vi "Set_Coupling.vi"(4 "Status":i32, 5 "error in (no error)":errorcluster, 6 "Set Coupling":u16(ring) items=["AC", "DC"], 7 "Choose_Device":T1(ring), 8 "Index":i32) -> (0 "error out":errorcluster, 1 "Status_out":i32, 2 "Device_type":T1(ring), 3 "Index_Out":i32)   [LabVIEW 2013, in "FEMTO_LUCI-10.lvlib"]
doc: "This function sets AC/DC coupling for the selected device."
uses:
  FEMTO_LUCI-10.lvlib
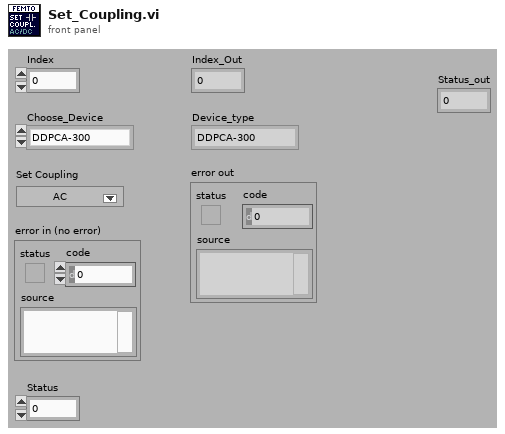
[diagram p1: front panel]
types:
  T1 = enum16{"DDPCA-300", "DLPCA-200", "DHPCA-100", "OE-200", "LIA-MV-150-S", "LIA-MV-150-D", "LIA-MV-200-L", "LIA-MV-200-H", "LIA-MVD-200-L", "LIA-MVD-200-H", "DLPVA-100-BUN-S", "DLPVA-100-BLN-S", "DLPVA-100-B-S", "DLPVA-100-B-D", "DLPVA-100-F-S", "DLPVA-100-F-D", "DHPVA-100", "DHPVA-200", "DUPVA-1-60", "DUPVA-1-70"}
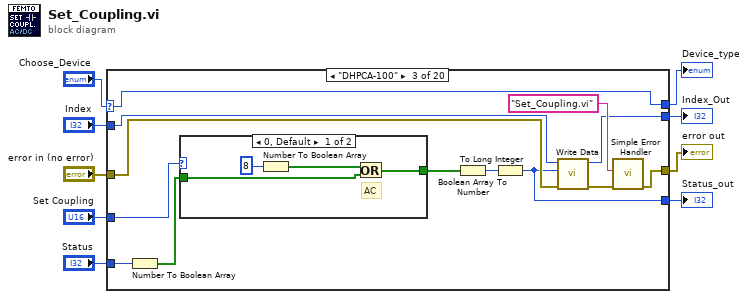
[diagram p0: block diagram]
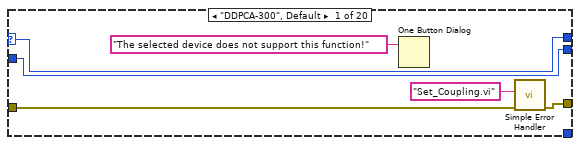
[diagram p2: hidden frame]
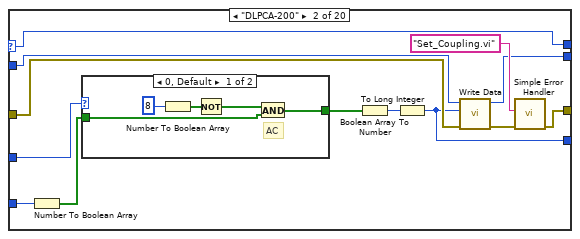
[diagram p3: hidden frame]
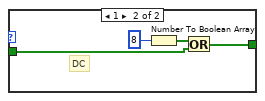
[diagram p4: hidden frame]
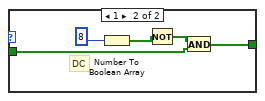
[diagram p5: hidden frame]
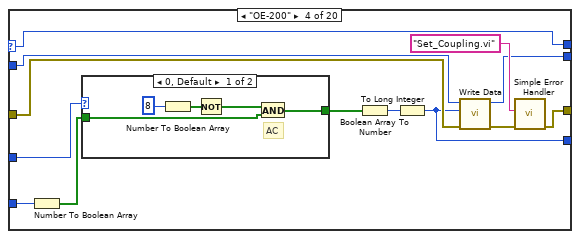
[diagram p6: hidden frame]
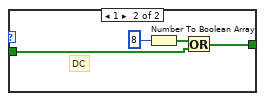
[diagram p7: hidden frame]
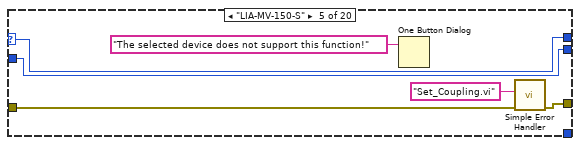
[diagram p8: hidden frame]
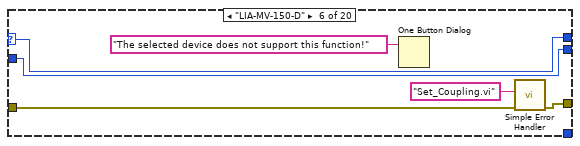
[diagram p9: hidden frame]
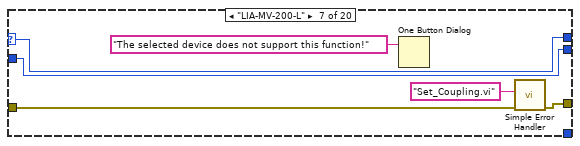
[diagram p10: hidden frame]
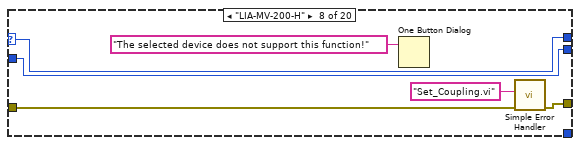
[diagram p11: hidden frame]
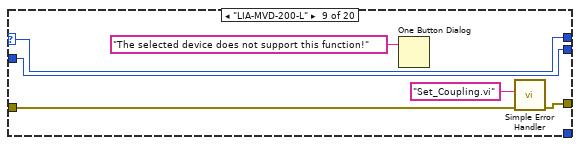
[diagram p12: hidden frame]
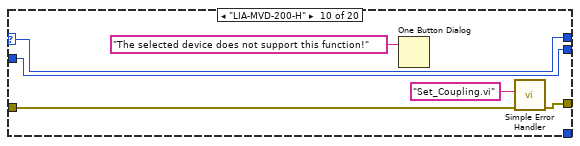
[diagram p13: hidden frame]
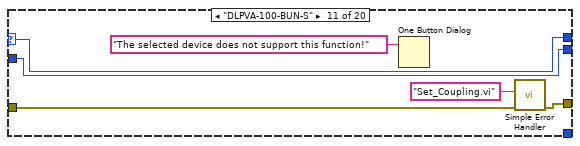
[diagram p14: hidden frame]
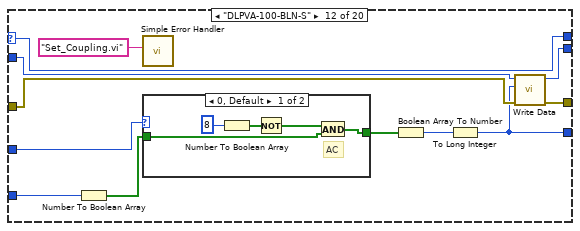
[diagram p15: hidden frame]
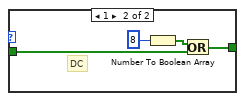
[diagram p16: hidden frame]
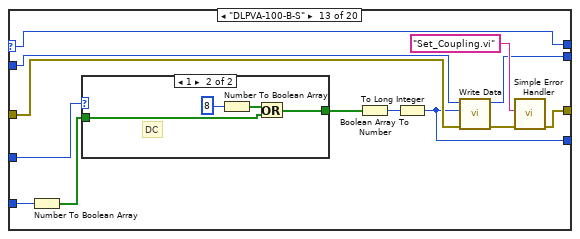
[diagram p17: hidden frame]
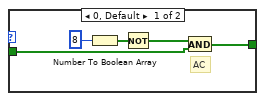
[diagram p18: hidden frame]
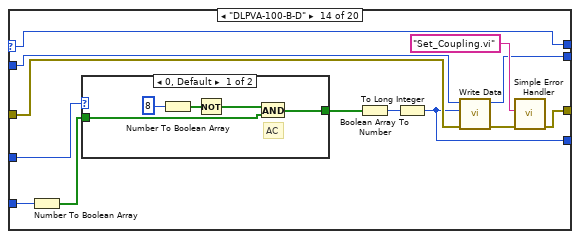
[diagram p19: hidden frame]
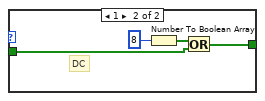
[diagram p20: hidden frame]
diagram:
  n1 = case shown="\"DHPCA-100\"" "Choose_Device" {
    selector: "Choose_Device" -> [w13 w27 w48 w70 w85 w91 w97 w103 w109 w115 w121 w134 w155 w172 w200 w221 w243 w265 w279 w285]
    tunnel: "error in (no error)" -> [w12 w18 w40 w62 w83 w89 w95 w102 w106 w112 w120 w130 w149 w174 w193 w215 w239 w261 w281 w287]
    tunnel: [w14 w28 w50 w71 w86 w92 w98 w104 w110 w116 w122 w129 w156 w178 w199 w222 w244 w266 w280 w286] -> w4
    tunnel: [w13 w27 w48 w70 w85 w91 w97 w103 w109 w115 w121 w134 w155 w172 w200 w221 w243 w265 w279 w285] -> w5
    tunnel: "Index" -> [w11 w20 w42 w64 w84 w90 w96 w101 w107 w114 w119 w128 w147 w171 w191 w213 w235 w259 w278 w284]
    tunnel: [w11 w19 w41 w63 w84 w90 w96 w101 w107 w114 w119 w127 w146 w170 w190 w212 w234 w258 w278 w284] -> w7
    tunnel: "Set Coupling" -> [_ w25 w43 w65 _ _ _ _ _ _ _ w125 w150 w168 w194 w216 w236 w256 _ _]
    tunnel: "Status" -> [_ w24 w44 w66 _ _ _ _ _ _ _ w126 w151 w169 w195 w217 w237 w257 _ _]
    tunnel: [_ w16 w38 w60 _ _ _ _ _ _ _ w124 w145 w167 w189 w211 w233 w255 _ _] -> w1
    frame "DDPCA-300", Default {
      n2 = One Button Dialog(message="The selected device does not support this function!") -> ()  [unwired: 2 out]
      n3 = call <vilib>:"Simple Error Handler.vi"("error source (\" \")"="Set_Coupling.vi" ("error source (\" \")"), "error in (no error)"=w12) -> ("error out"=w14:errorcluster)  [unwired: 1 in, 6 out]
    }
    frame "DLPCA-200" {
      n4 = Number To Boolean Array(number=w24) -> (Boolean array=w23:bool[])
      n5 = case shown="0, Default" w25 {
        tunnel: w23 -> [w30 w35]
        tunnel: [w29 w34] -> w21
        frame 0, Default {
          # "AC"
          n6 = Number To Boolean Array(number=8 ("x")) -> (Boolean array=w32:bool[])
          n7 = Not(x=w32) -> (.not. x?=w33:bool[])
          n8 = And(x=w33, y=w30) -> (x .and. y?=w29:bool[])
        }
        frame 1 {
          # "DC"
          n9 = Number To Boolean Array(number=8) -> (Boolean array=w37:bool[])
          n10 = Or(x=w37, y=w35) -> (x .or. y?=w34:bool[])
        }
      }
      n11 = Boolean Array To Number(Boolean array=w21) -> (number=w22:u32)
      n12 = To Long Integer(number=w22) -> (32bit integer=w16:i32)
      n13 = call "Write Data.vi"("error in (no error)"=w18, "data_low"=w16, "index"=w20) -> ("error out"=w17:errorcluster, "index_out"=w19:i32)  [unwired: 1 in, 6 out]
      n14 = call <vilib>:"Simple Error Handler.vi"("error source (\" \")"="Set_Coupling.vi" ("error source (\" \")"), "error in (no error)"=w17) -> ("error out"=w28:errorcluster)  [unwired: 1 in, 6 out]
    }
    frame "DHPCA-100" {
      n15 = Number To Boolean Array(number=w44) -> (Boolean array=w47:bool[])
      n16 = case shown="0, Default" w43 {
        tunnel: w47 -> [w53 w58]
        tunnel: [w52 w57] -> w45
        frame 0, Default {
          # "AC"
          n17 = Number To Boolean Array(number=8 ("x")) -> (Boolean array=w51:bool[])
          n18 = Or(x=w51, y=w53) -> (x .or. y?=w52:bool[])
        }
        frame 1 {
          # "DC"
          n19 = Number To Boolean Array(number=8) -> (Boolean array=w56:bool[])
          n20 = Not(x=w56) -> (.not. x?=w55:bool[])
          n21 = And(x=w55, y=w58) -> (x .and. y?=w57:bool[])
        }
      }
      n22 = Boolean Array To Number(Boolean array=w45) -> (number=w46:u32)
      n23 = To Long Integer(number=w46) -> (32bit integer=w38:i32)
      n24 = call "Write Data.vi"("error in (no error)"=w40, "data_low"=w38, "index"=w42) -> ("error out"=w39:errorcluster, "index_out"=w41:i32)  [unwired: 1 in, 6 out]
      n25 = call <vilib>:"Simple Error Handler.vi"("error source (\" \")"="Set_Coupling.vi" ("error source (\" \")"), "error in (no error)"=w39) -> ("error out"=w50:errorcluster)  [unwired: 1 in, 6 out]
    }
    frame "OE-200" {
      n26 = Number To Boolean Array(number=w66) -> (Boolean array=w69:bool[])
      n27 = case shown="0, Default" w65 {
        tunnel: w69 -> [w74 w79]
        tunnel: [w73 w78] -> w67
        frame 0, Default {
          # "AC"
          n28 = Number To Boolean Array(number=8 ("x")) -> (Boolean array=w76:bool[])
          n29 = Not(x=w76) -> (.not. x?=w77:bool[])
          n30 = And(x=w77, y=w74) -> (x .and. y?=w73:bool[])
        }
        frame 1 {
          # "DC"
          n31 = Number To Boolean Array(number=8) -> (Boolean array=w81:bool[])
          n32 = Or(x=w81, y=w79) -> (x .or. y?=w78:bool[])
        }
      }
      n33 = Boolean Array To Number(Boolean array=w67) -> (number=w68:u32)
      n34 = To Long Integer(number=w68) -> (32bit integer=w60:i32)
      n35 = call "Write Data.vi"("error in (no error)"=w62, "data_low"=w60, "index"=w64) -> ("error out"=w61:errorcluster, "index_out"=w63:i32)  [unwired: 1 in, 6 out]
      n36 = call <vilib>:"Simple Error Handler.vi"("error source (\" \")"="Set_Coupling.vi" ("error source (\" \")"), "error in (no error)"=w61) -> ("error out"=w71:errorcluster)  [unwired: 1 in, 6 out]
    }
    frame "LIA-MV-150-S" {
      n37 = One Button Dialog(message="The selected device does not support this function!") -> ()  [unwired: 2 out]
      n38 = call <vilib>:"Simple Error Handler.vi"("error source (\" \")"="Set_Coupling.vi" ("error source (\" \")"), "error in (no error)"=w83) -> ("error out"=w86:errorcluster)  [unwired: 1 in, 6 out]
    }
    frame "LIA-MV-150-D" {
      n39 = One Button Dialog(message="The selected device does not support this function!") -> ()  [unwired: 2 out]
      n40 = call <vilib>:"Simple Error Handler.vi"("error source (\" \")"="Set_Coupling.vi" ("error source (\" \")"), "error in (no error)"=w89) -> ("error out"=w92:errorcluster)  [unwired: 1 in, 6 out]
    }
    frame "LIA-MV-200-L" {
      n41 = One Button Dialog(message="The selected device does not support this function!") -> ()  [unwired: 2 out]
      n42 = call <vilib>:"Simple Error Handler.vi"("error source (\" \")"="Set_Coupling.vi" ("error source (\" \")"), "error in (no error)"=w95) -> ("error out"=w98:errorcluster)  [unwired: 1 in, 6 out]
    }
    frame "LIA-MV-200-H" {
      n43 = One Button Dialog(message="The selected device does not support this function!") -> ()  [unwired: 2 out]
      n44 = call <vilib>:"Simple Error Handler.vi"("error source (\" \")"="Set_Coupling.vi" ("error source (\" \")"), "error in (no error)"=w102) -> ("error out"=w104:errorcluster)  [unwired: 1 in, 6 out]
    }
    frame "LIA-MVD-200-L" {
      n45 = One Button Dialog(message="The selected device does not support this function!") -> ()  [unwired: 2 out]
      n46 = call <vilib>:"Simple Error Handler.vi"("error source (\" \")"="Set_Coupling.vi" ("error source (\" \")"), "error in (no error)"=w106) -> ("error out"=w110:errorcluster)  [unwired: 1 in, 6 out]
    }
    frame "LIA-MVD-200-H" {
      n47 = One Button Dialog(message="The selected device does not support this function!") -> ()  [unwired: 2 out]
      n48 = call <vilib>:"Simple Error Handler.vi"("error source (\" \")"="Set_Coupling.vi" ("error source (\" \")"), "error in (no error)"=w112) -> ("error out"=w116:errorcluster)  [unwired: 2 in, 5 out]
    }
    frame "DLPVA-100-BUN-S" {
      n49 = One Button Dialog(message="The selected device does not support this function!") -> ()  [unwired: 2 out]
      n50 = call <vilib>:"Simple Error Handler.vi"("error source (\" \")"="Set_Coupling.vi" ("error source (\" \")"), "error in (no error)"=w120) -> ("error out"=w122:errorcluster)  [unwired: 1 in, 6 out]
    }
    frame "DLPVA-100-BLN-S" {
      n51 = Number To Boolean Array(number=w126) -> (Boolean array=w133:bool[])
      n52 = call <vilib>:"Simple Error Handler.vi"("error source (\" \")"="Set_Coupling.vi" ("error source (\" \")")) -> ()  [unwired: 2 in, 7 out]
      n53 = case shown="0, Default" w125 {
        tunnel: w133 -> [w137 w142]
        tunnel: [w136 w141] -> w131
        frame 0, Default {
          # "AC"
          n54 = Number To Boolean Array(number=8 ("x")) -> (Boolean array=w139:bool[])
          n55 = Not(x=w139) -> (.not. x?=w140:bool[])
          n56 = And(x=w140, y=w137) -> (x .and. y?=w136:bool[])
        }
        frame 1 {
          # "DC"
          n57 = Number To Boolean Array(number=8) -> (Boolean array=w144:bool[])
          n58 = Or(x=w144, y=w142) -> (x .or. y?=w141:bool[])
        }
      }
      n59 = Boolean Array To Number(Boolean array=w131) -> (number=w132:u32)
      n60 = To Long Integer(number=w132) -> (32bit integer=w124:i32)
      n61 = call "Write Data.vi"("error in (no error)"=w130, "data_low"=w124, "index"=w128) -> ("error out"=w129:errorcluster, "index_out"=w127:i32)  [unwired: 1 in, 6 out]
    }
    frame "DLPVA-100-B-S" {
      n62 = Number To Boolean Array(number=w151) -> (Boolean array=w154:bool[])
      n63 = case shown="1" w150 {
        tunnel: w154 -> [w159 w164]
        tunnel: [w158 w163] -> w152
        frame 0, Default {
          # "AC"
          n64 = Number To Boolean Array(number=8 ("x")) -> (Boolean array=w161:bool[])
          n65 = Not(x=w161) -> (.not. x?=w162:bool[])
          n66 = And(x=w162, y=w159) -> (x .and. y?=w158:bool[])
        }
        frame 1 {
          # "DC"
          n67 = Number To Boolean Array(number=8) -> (Boolean array=w166:bool[])
          n68 = Or(x=w166, y=w164) -> (x .or. y?=w163:bool[])
        }
      }
      n69 = Boolean Array To Number(Boolean array=w152) -> (number=w153:u32)
      n70 = To Long Integer(number=w153) -> (32bit integer=w145:i32)
      n71 = call "Write Data.vi"("error in (no error)"=w149, "data_low"=w145, "index"=w147) -> ("error out"=w148:errorcluster, "index_out"=w146:i32)  [unwired: 1 in, 6 out]
      n72 = call <vilib>:"Simple Error Handler.vi"("error source (\" \")"="Set_Coupling.vi" ("error source (\" \")"), "error in (no error)"=w148) -> ("error out"=w156:errorcluster)  [unwired: 1 in, 6 out]
    }
    frame "DLPVA-100-B-D" {
      n73 = Number To Boolean Array(number=w169) -> (Boolean array=w177:bool[])
      n74 = case shown="0, Default" w168 {
        tunnel: w177 -> [w181 w186]
        tunnel: [w180 w185] -> w175
        frame 0, Default {
          # "AC"
          n75 = Number To Boolean Array(number=8 ("x")) -> (Boolean array=w183:bool[])
          n76 = Not(x=w183) -> (.not. x?=w184:bool[])
          n77 = And(x=w184, y=w181) -> (x .and. y?=w180:bool[])
        }
        frame 1 {
          # "DC"
          n78 = Number To Boolean Array(number=8) -> (Boolean array=w188:bool[])
          n79 = Or(x=w188, y=w186) -> (x .or. y?=w185:bool[])
        }
      }
      n80 = Boolean Array To Number(Boolean array=w175) -> (number=w176:u32)
      n81 = To Long Integer(number=w176) -> (32bit integer=w167:i32)
      n82 = call "Write Data.vi"("error in (no error)"=w174, "data_low"=w167, "index"=w171) -> ("error out"=w173:errorcluster, "index_out"=w170:i32)  [unwired: 1 in, 6 out]
      n83 = call <vilib>:"Simple Error Handler.vi"("error source (\" \")"="Set_Coupling.vi" ("error source (\" \")"), "error in (no error)"=w173) -> ("error out"=w178:errorcluster)  [unwired: 1 in, 6 out]
    }
    frame "DLPVA-100-F-S" {
      n84 = Number To Boolean Array(number=w195) -> (Boolean array=w198:bool[])
      n85 = case shown="0, Default" w194 {
        tunnel: w198 -> [w203 w208]
        tunnel: [w202 w207] -> w196
        frame 0, Default {
          # "AC"
          n86 = Number To Boolean Array(number=8 ("x")) -> (Boolean array=w205:bool[])
          n87 = Not(x=w205) -> (.not. x?=w206:bool[])
          n88 = And(x=w206, y=w203) -> (x .and. y?=w202:bool[])
        }
        frame 1 {
          # "DC"
          n89 = Number To Boolean Array(number=8) -> (Boolean array=w210:bool[])
          n90 = Or(x=w210, y=w208) -> (x .or. y?=w207:bool[])
        }
      }
      n91 = Boolean Array To Number(Boolean array=w196) -> (number=w197:u32)
      n92 = To Long Integer(number=w197) -> (32bit integer=w189:i32)
      n93 = call "Write Data.vi"("error in (no error)"=w193, "data_low"=w189, "index"=w191) -> ("error out"=w192:errorcluster, "index_out"=w190:i32)  [unwired: 1 in, 6 out]
      n94 = call <vilib>:"Simple Error Handler.vi"("error source (\" \")"="Set_Coupling.vi" ("error source (\" \")"), "error in (no error)"=w192) -> ("error out"=w199:errorcluster)  [unwired: 1 in, 6 out]
    }
    frame "DLPVA-100-F-D" {
      n95 = Number To Boolean Array(number=w217) -> (Boolean array=w220:bool[])
      n96 = case shown="1" w216 {
        tunnel: w220 -> [w225 w230]
        tunnel: [w224 w229] -> w218
        frame 0, Default {
          # "AC"
          n97 = Number To Boolean Array(number=8 ("x")) -> (Boolean array=w227:bool[])
          n98 = Not(x=w227) -> (.not. x?=w228:bool[])
          n99 = And(x=w228, y=w225) -> (x .and. y?=w224:bool[])
        }
        frame 1 {
          # "DC"
          n100 = Number To Boolean Array(number=8) -> (Boolean array=w232:bool[])
          n101 = Or(x=w232, y=w230) -> (x .or. y?=w229:bool[])
        }
      }
      n102 = Boolean Array To Number(Boolean array=w218) -> (number=w219:u32)
      n103 = To Long Integer(number=w219) -> (32bit integer=w211:i32)
      n104 = call "Write Data.vi"("error in (no error)"=w215, "data_low"=w211, "index"=w213) -> ("error out"=w214:errorcluster, "index_out"=w212:i32)  [unwired: 1 in, 6 out]
      n105 = call <vilib>:"Simple Error Handler.vi"("error source (\" \")"="Set_Coupling.vi" ("error source (\" \")"), "error in (no error)"=w214) -> ("error out"=w222:errorcluster)  [unwired: 1 in, 6 out]
    }
    frame "DHPVA-100" {
      n106 = Number To Boolean Array(number=w237) -> (Boolean array=w242:bool[])
      n107 = case shown="0, Default" w236 {
        tunnel: w242 -> [w247 w252]
        tunnel: [w246 w251] -> w240
        frame 0, Default {
          # "AC"
          n108 = Number To Boolean Array(number=8 ("x")) -> (Boolean array=w249:bool[])
          n109 = Not(x=w249) -> (.not. x?=w250:bool[])
          n110 = And(x=w250, y=w247) -> (x .and. y?=w246:bool[])
        }
        frame 1 {
          # "DC"
          n111 = Number To Boolean Array(number=8) -> (Boolean array=w254:bool[])
          n112 = Or(x=w254, y=w252) -> (x .or. y?=w251:bool[])
        }
      }
      n113 = Boolean Array To Number(Boolean array=w240) -> (number=w241:u32)
      n114 = To Long Integer(number=w241) -> (32bit integer=w233:i32)
      n115 = call "Write Data.vi"("error in (no error)"=w239, "data_low"=w233, "index"=w235) -> ("error out"=w238:errorcluster, "index_out"=w234:i32)  [unwired: 1 in, 6 out]
      n116 = call <vilib>:"Simple Error Handler.vi"("error source (\" \")"="Set_Coupling.vi" ("error source (\" \")"), "error in (no error)"=w238) -> ("error out"=w244:errorcluster)  [unwired: 1 in, 6 out]
    }
    frame "DHPVA-200" {
      n117 = Number To Boolean Array(number=w257) -> (Boolean array=w264:bool[])
      n118 = case shown="0, Default" w256 {
        tunnel: w264 -> [w269 w274]
        tunnel: [w268 w273] -> w262
        frame 0, Default {
          # "AC"
          n119 = Number To Boolean Array(number=8 ("x")) -> (Boolean array=w271:bool[])
          n120 = Not(x=w271) -> (.not. x?=w272:bool[])
          n121 = And(x=w272, y=w269) -> (x .and. y?=w268:bool[])
        }
        frame 1 {
          # "DC"
          n122 = Number To Boolean Array(number=8) -> (Boolean array=w276:bool[])
          n123 = Or(x=w276, y=w274) -> (x .or. y?=w273:bool[])
        }
      }
      n124 = Boolean Array To Number(Boolean array=w262) -> (number=w263:u32)
      n125 = To Long Integer(number=w263) -> (32bit integer=w255:i32)
      n126 = call "Write Data.vi"("error in (no error)"=w261, "data_low"=w255, "index"=w259) -> ("error out"=w260:errorcluster, "index_out"=w258:i32)  [unwired: 1 in, 6 out]
      n127 = call <vilib>:"Simple Error Handler.vi"("error source (\" \")"="Set_Coupling.vi" ("error source (\" \")"), "error in (no error)"=w260) -> ("error out"=w266:errorcluster)  [unwired: 1 in, 6 out]
    }
    frame "DUPVA-1-60" {
      n128 = One Button Dialog(message="The selected device does not support this function!") -> ()  [unwired: 2 out]
      n129 = call <vilib>:"Simple Error Handler.vi"("error source (\" \")"="Set_Coupling.vi" ("error source (\" \")"), "error in (no error)"=w281) -> ("error out"=w280:errorcluster)  [unwired: 1 in, 6 out]
    }
    frame "DUPVA-1-70" {
      n130 = One Button Dialog(message="The selected device does not support this function!") -> ()  [unwired: 2 out]
      n131 = call <vilib>:"Simple Error Handler.vi"("error source (\" \")"="Set_Coupling.vi" ("error source (\" \")"), "error in (no error)"=w287) -> ("error out"=w286:errorcluster)  [unwired: 1 in, 6 out]
    }
  }
  "error out" <- w4
  "Device_type" <- w5
  "Index_Out" <- w7
  "Status_out" <- w1
